vi "stopDriveMode.vi"() -> ()   [LabVIEW 2018, in "MotorControllerClass.lvclass"]
uses:
  BMS/MotorControllerClass.lvclass
panel:
  out "MotorControllerClass out":refnum<class "MotorControllerClass.lvclass">
  in  "MotorControllerClass in":refnum<class "MotorControllerClass.lvclass">
  out "interface object out":refnum<k20>
  in  "interface object in":refnum<k20>
  out "stopDriveRes":u32
  out "error out":errorcluster
  in  "error in (no error)":errorcluster
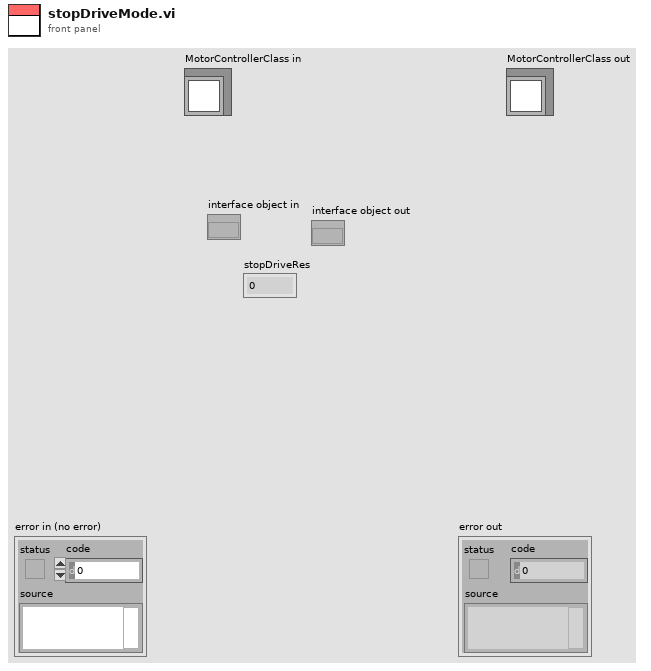
[diagram p1: front panel]
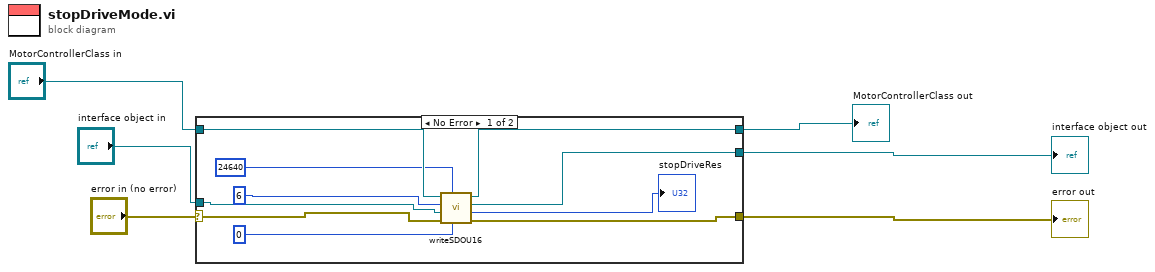
[diagram p0: block diagram]
diagram:
  n1 = case shown="No Error" "error in (no error)" {
    selector: "error in (no error)" -> [w11 w19]
    tunnel: [w9 w19] -> w5
    tunnel: "interface object in" -> [w12 w18]
    tunnel: [w7 w18] -> w3
    tunnel: "MotorControllerClass in" -> [w16 w17]
    tunnel: [w15 w17] -> w1
    frame No Error {
      n2 = call "writeSDOU16.vi"("object sub-index (0)"=u8 0, "object index"=u16 24640, "error in (no error)"=w11, "interface object in"=w12, "inputNumber"=u16 6, "MotorControllerClass in"=w16) -> ("error out"=w9:errorcluster, "completion code"=→"stopDriveRes":u32, "interface object out"=w7:refnum<k20>, "MotorControllerClass out"=w15:refnum<class "MotorControllerClass.lvclass">)  [unwired: 2 in]
    }
    frame Error {
    }
  }
  "error out" <- w5
  "interface object out" <- w3
  "MotorControllerClass out" <- w1
